vi "ForwardMultiply.vi"(10 "Inputs":dbl[](array[numeric]), 11 "Neuron Stucture In":T1) -> (2 "Outputs":dbl[](array[numeric]), 3 "Neuron Stucture Out":T1)   [LabVIEW 2012]
uses:
  NeuronData.ctl
panel:
  # "Chuck Streb Dec2007"
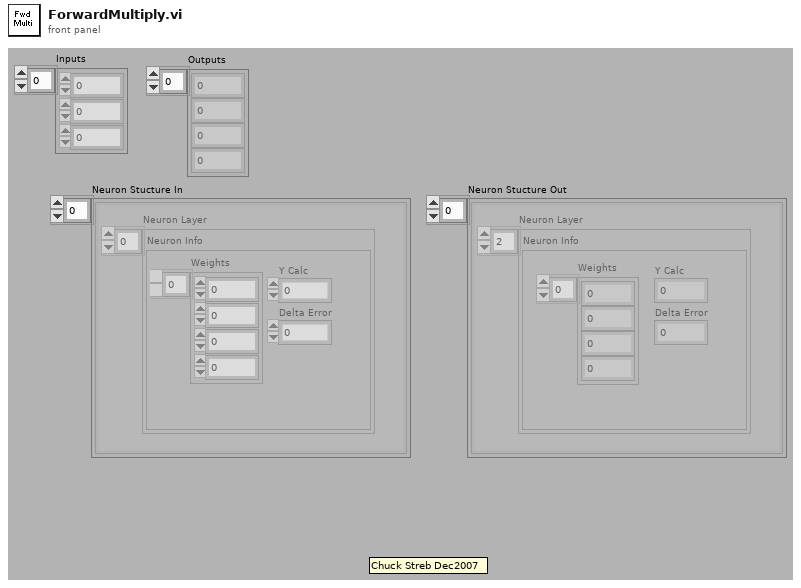
[diagram p1: front panel]
types:
  T1 = typedef "NeuronData.ctl" = cluster{"Neuron Layer":cluster{"Weights":dbl[], "Y Calc":dbl, "Delta Error":dbl}[]}[]
  T2 = cluster{"Weights":dbl[], "Y Calc":dbl, "Delta Error":dbl}[]
  T3 = cluster{"Weights":dbl[], "Y Calc":dbl, "Delta Error":dbl}
  T4 = cluster{"Neuron Layer":cluster{"Weights":dbl[], "Y Calc":dbl, "Delta Error":dbl}[]}
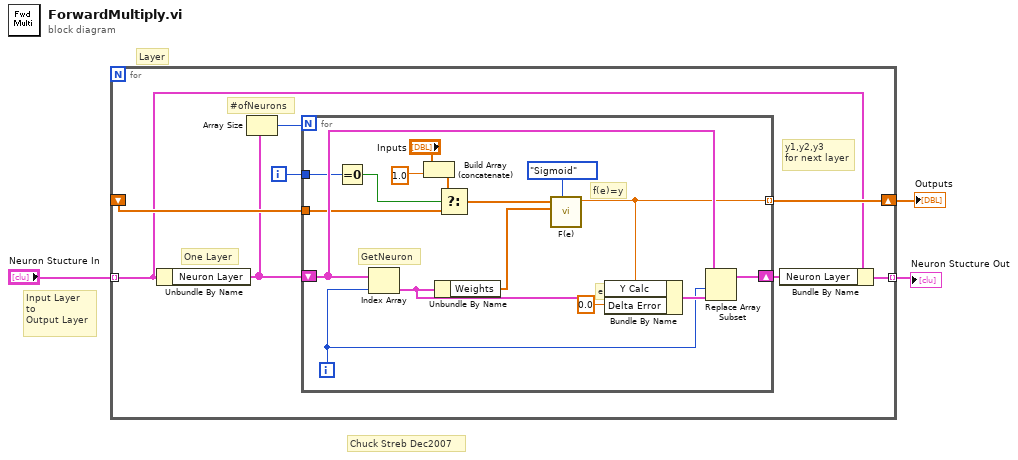
[diagram p0: block diagram]
diagram:
  # "Chuck Streb Dec2007"
  # "Layer"
  # "Input Layer\nto\nOutput Layer"
  n1 = for {
    tunnel: "Neuron Stucture In" -> [w6] mode=indexing
    shift-right: [w9] -> w2
    shift-left: _ -> [w8]
    tunnel: [w4] -> w1 mode=indexing
    i -> [w10]
    # "y1,y2,y3\nfor next layer"
    # "One Layer"
    # "#ofNeurons"
    n2 = Unbundle By Name(w6) -> ("Neuron Layer"=w7:T2)
    n3 = Array Size(array=w7) -> (size(s)=w11:i32)
    n4 = for {
      N: w11 -> [_]
      shift-right: [w26] -> w5
      shift-left: w7 -> [w24]
      tunnel: w10 -> [w21]
      tunnel: [w17] -> w9 mode=indexing
      tunnel: w8 -> [w19]
      i -> [w25]
      # "f(e)=y"
      # "e"
      # "GetNeuron"
      n5 = Equal To 0?(x=w21) -> (x = 0?=w20:bool)
      n6 = Index Array(array=w24, index=w25) -> (element=w23:T3)
      n7 = Build Array (concatenate)("Inputs", 1.0) -> (w12:dbl[])
      n8 = Unbundle By Name(w23) -> ("Weights"=w18:dbl[])
      n9 = Select(t=w12, s=w20, f=w19) -> (s? t:f=w14:dbl[])
      n10 = call "F(e).vi"("Neuron Type"=enum16{"Linear", "Sigmoid", "Tangent hyp."}."Sigmoid", "Weights"=w18, "Inputs"=w14) -> ("f(e)"=w17:dbl)  [unwired: 8 in]
      n11 = Bundle By Name(cluster=w23, "Y Calc"=w17, "Delta Error"=0.0) -> (w27:T3)
      n12 = Replace Array Subset(array=w24, new element=w27, index=w25) -> (w26:T2)
    }
    n13 = Bundle By Name(cluster=w6, "Neuron Layer"=w5) -> (w4:T4)
  }
  "Outputs" <- w2
  "Neuron Stucture Out" <- w1
